vi "CTRE_Phoenix_CANdle_HasResetOccurred.vi"(8 "error in":errorcluster, 11 "CTRE_CANdle_DeviceRef":T1) -> (0 "error out":errorcluster, 2 "Has Reset Occurred?":bool, 3 "CTRE_CANdle_DeviceRef":T1)   [LabVIEW 2020]
doc: "Returns TRUE if the device has had a reset occur since the last call."
uses:
  <vilib>/Rock Robotics/WPI/ThirdParty/Phoenix-LabVIEW/CANdle/Controls/CTRE_Phoenix_CANdle_DeviceRef.ctl
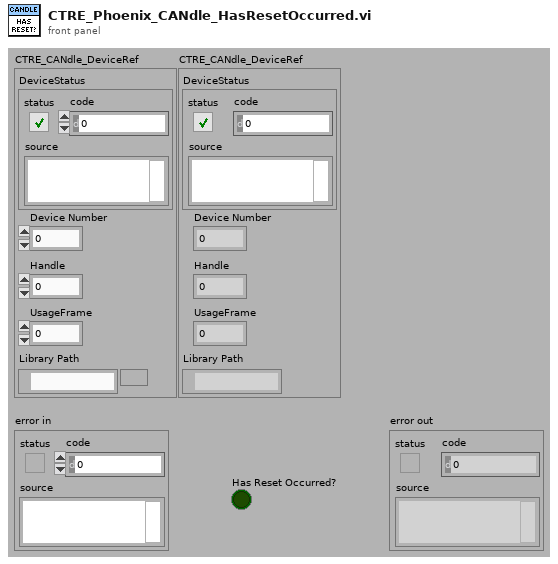
[diagram p1: front panel]
types:
  T1 = typedef "CTRE_Phoenix_CANdle_DeviceRef.ctl" = cluster{"DeviceStatus":errorcluster, "Device Number":u8, "Handle":u64, "UsageFrame":u32, "Library Path":path}
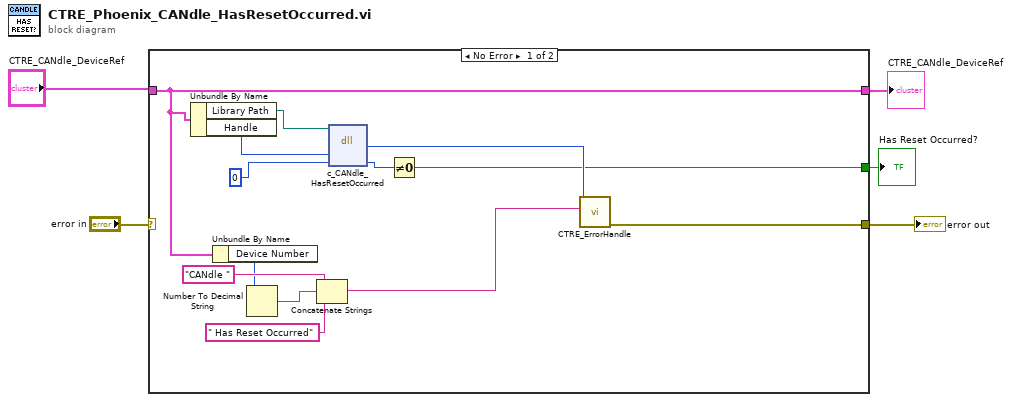
[diagram p0: block diagram]
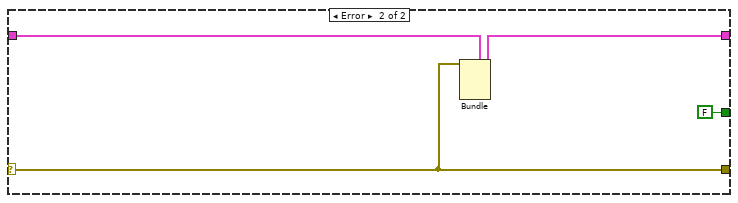
[diagram p2: hidden frame]
diagram:
  n1 = case shown="No Error" "error in" {
    selector: "error in" -> [_ w21]
    tunnel: "CTRE_CANdle_DeviceRef" -> [w10 w22]
    tunnel: [w17 w21] -> w5
    tunnel: [w10 w20] -> w1
    tunnel: [w6 FALSE] -> w3
    frame No Error {
      n2 = Unbundle By Name(w10) -> ("Library Path"=w9:path, "Handle"=w8:u64)
      n3 = Unbundle By Name(w10) -> ("Device Number"=w13:u8)
      n4 = Number To Decimal String(number=w13) -> (decimal integer string=w15:string)  [unwired: 1 in]
      n5 = Concatenate Strings("CANdle " ("string"), w15, " Has Reset Occurred" ("string")) -> (w11:string)
      n6 = dll-call lib="?" fn="c_CANdle_HasResetOccurred"(path in=w9, "handle"=w8, "hasResetOccurred"=u32 0 ("appliedThrottle")) -> ("return type"=w12:i32, "hasResetOccurred"=w7:u8)  [unwired: 3 in, 2 out]
      n7 = Not Equal To 0?(x=w7) -> (x != 0?=w6:bool)
      n8 = call <vilib>:"CTRE_ErrorHandle.vi"("origin"=w11, "code"=w12) -> ("error out"=w17:errorcluster)  [unwired: 9 in]
    }
    frame Error {
      n9 = Bundle(cluster=w22, "DeviceStatus"=w21) -> (w20:T1)  [unwired: 4 in]
    }
  }
  "error out" <- w5
  "Has Reset Occurred?" <- w3
  "CTRE_CANdle_DeviceRef" <- w1
